vi "Item Setting.vi"(3 "error in":errorcluster) -> (0 "error out":errorcluster)   [LabVIEW 2020]
panel:
  in  "Edit Button":bool
  in  "Delete Button":bool
  in  "Add Button":bool
  in  "Items":i32(listbox)
  in  "Exit Button":bool
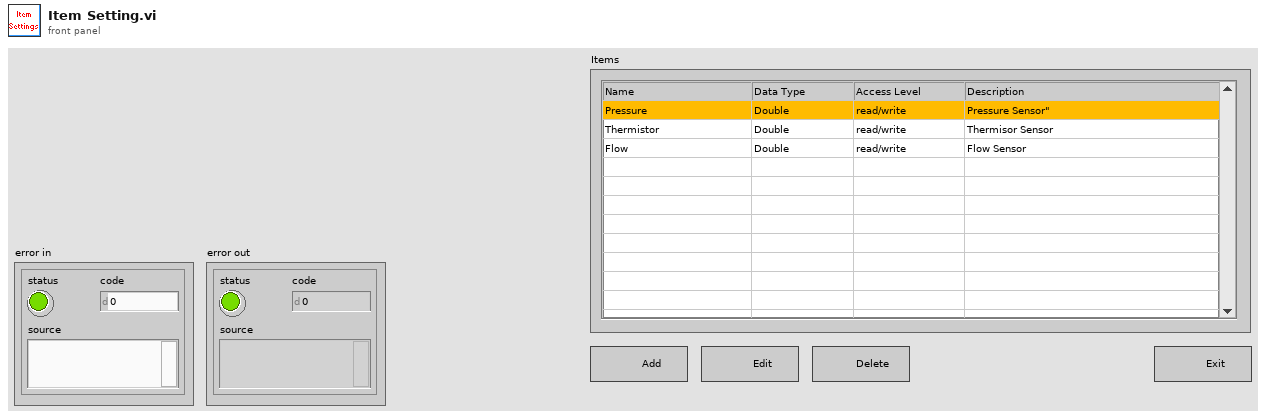
[diagram p1: front panel]
types:
  T1 = cluster{"Name":string, "Data type":u16, "Access level":u16, "Description":string}[]
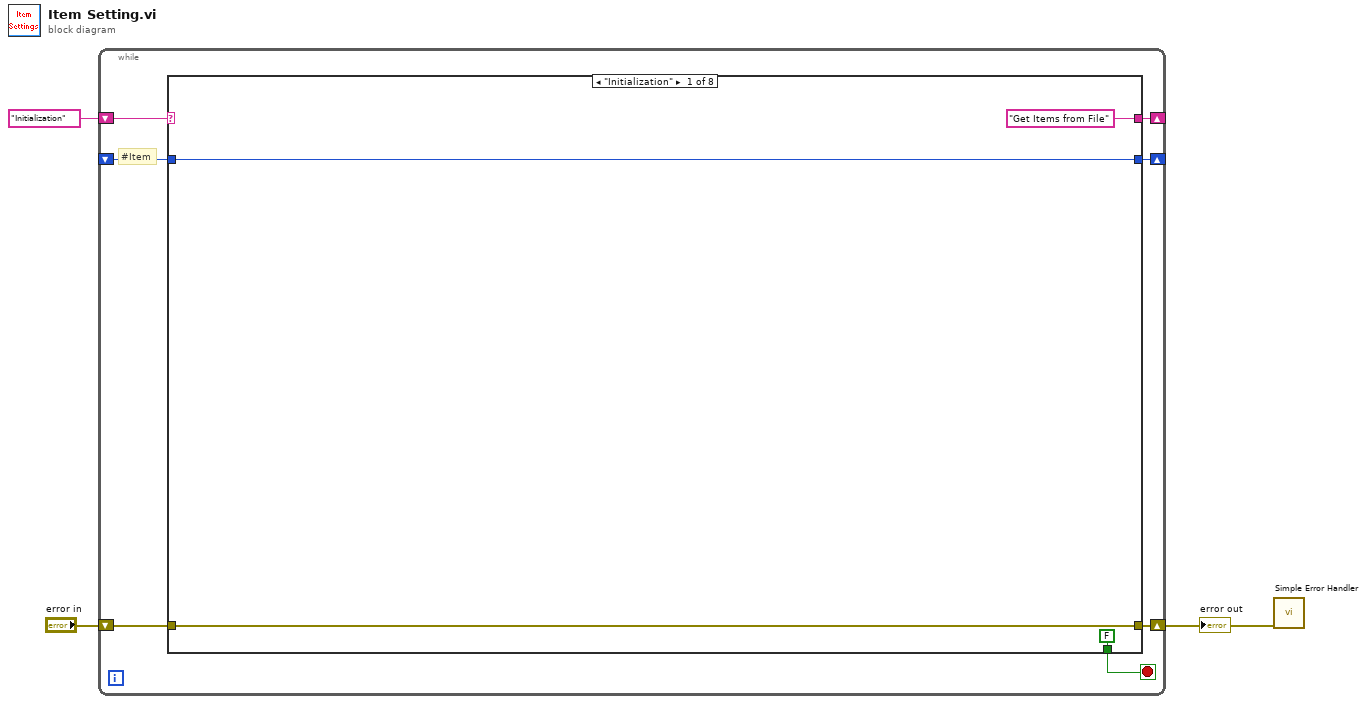
[diagram p0: block diagram]
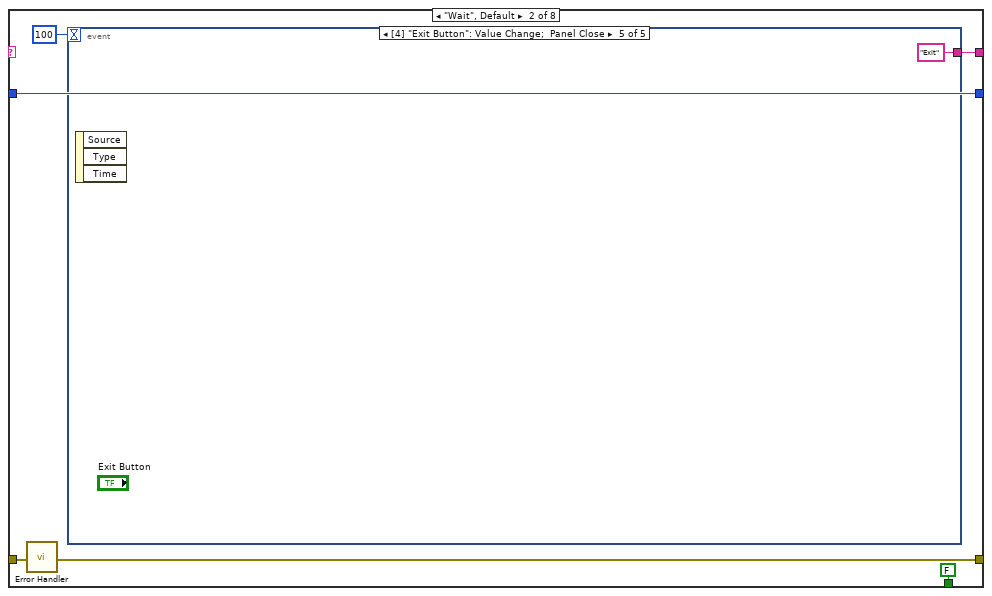
[diagram p2: hidden frame]
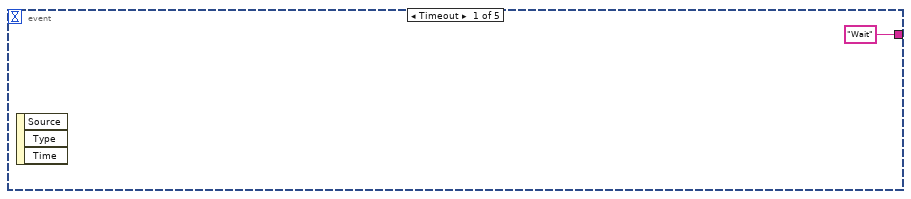
[diagram p3: hidden frame]
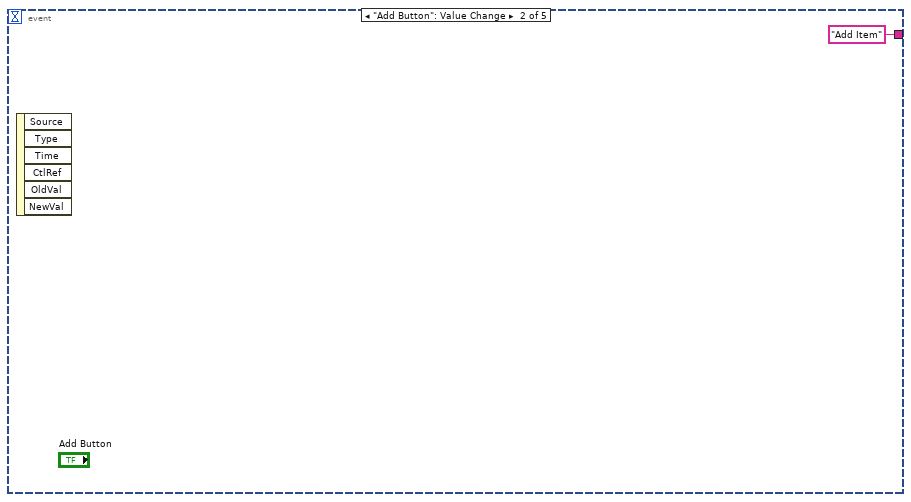
[diagram p4: hidden frame]
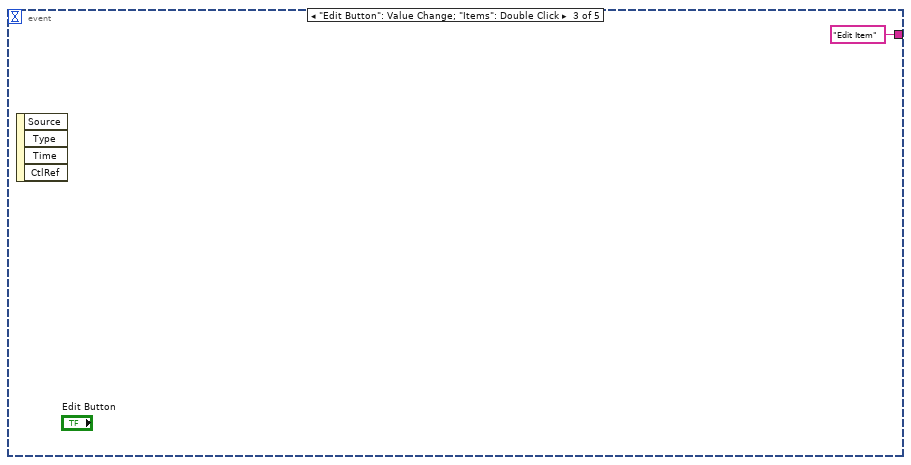
[diagram p5: hidden frame]
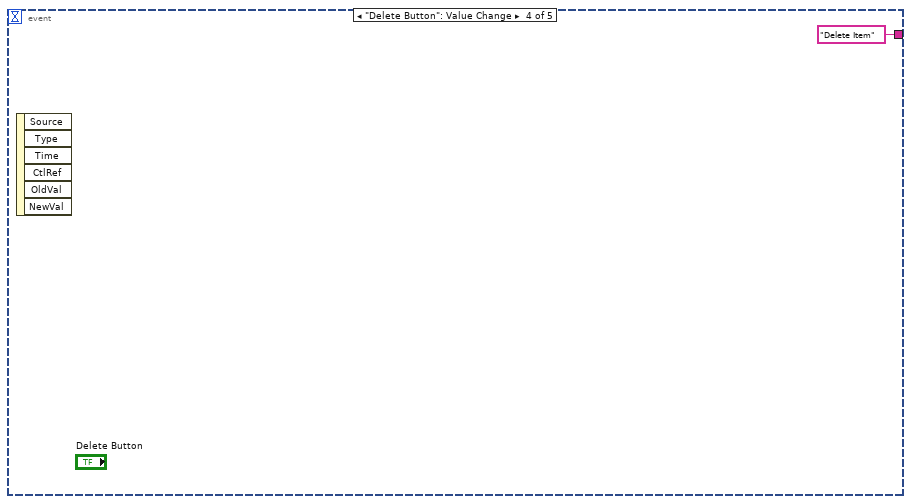
[diagram p6: hidden frame]
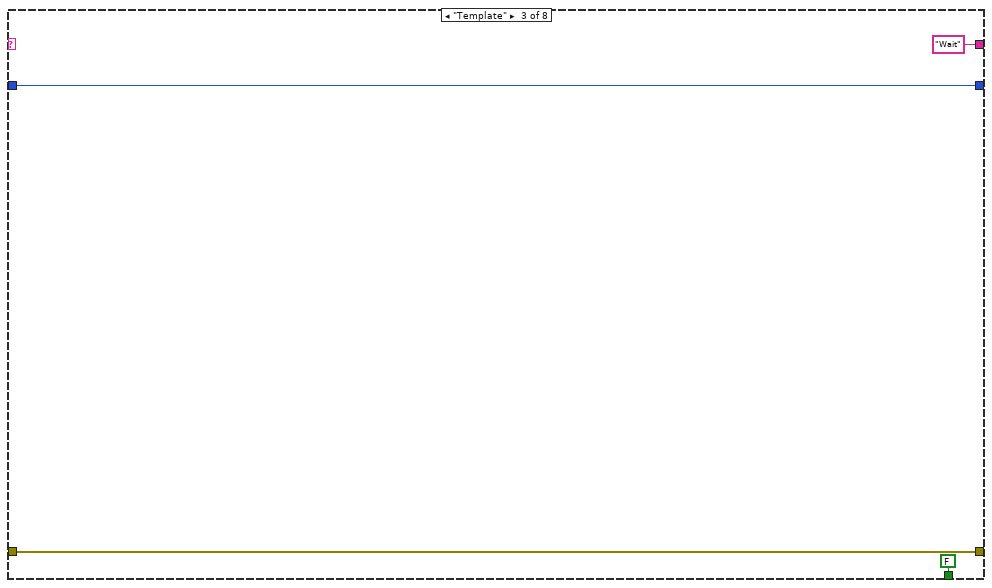
[diagram p7: hidden frame]
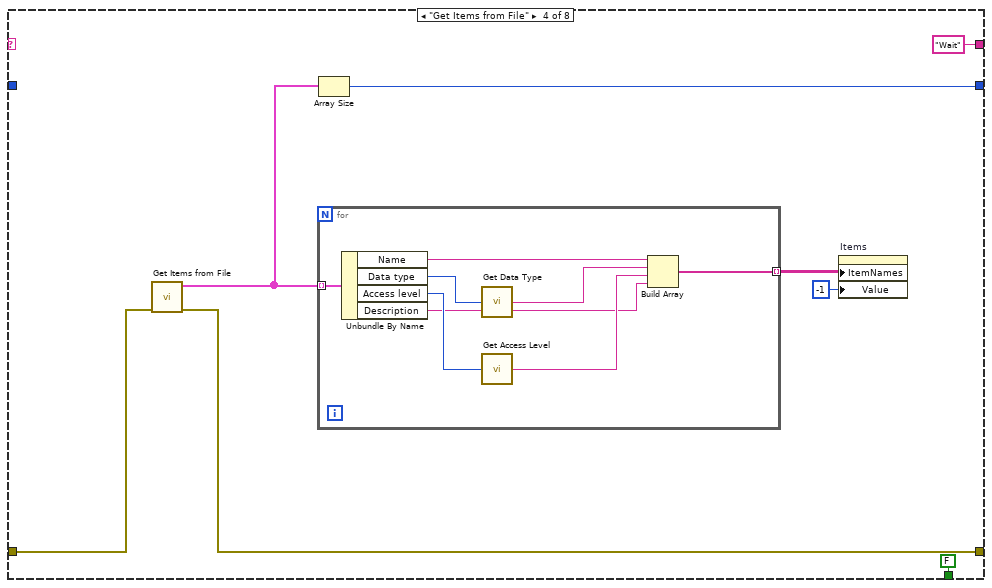
[diagram p8: hidden frame]
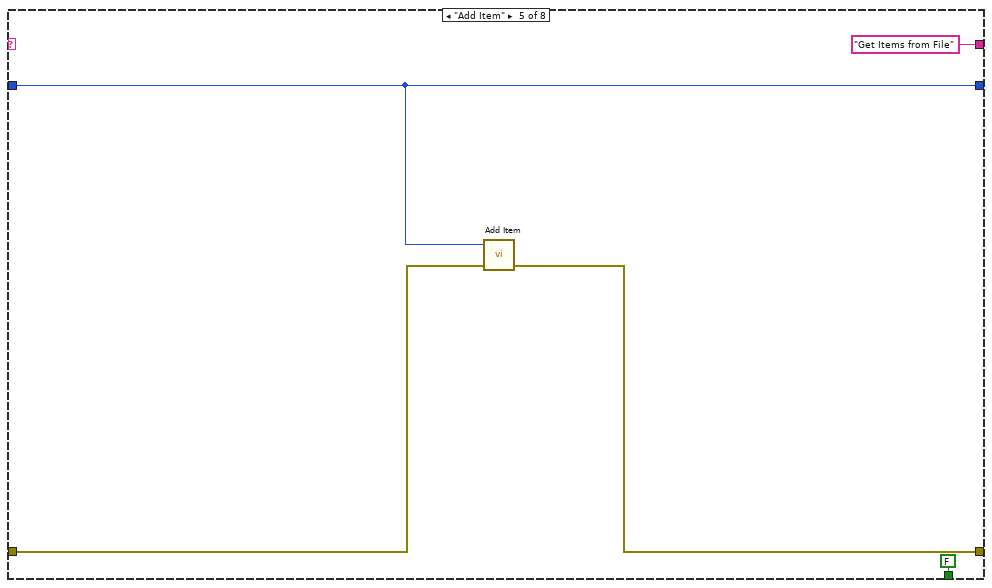
[diagram p9: hidden frame]
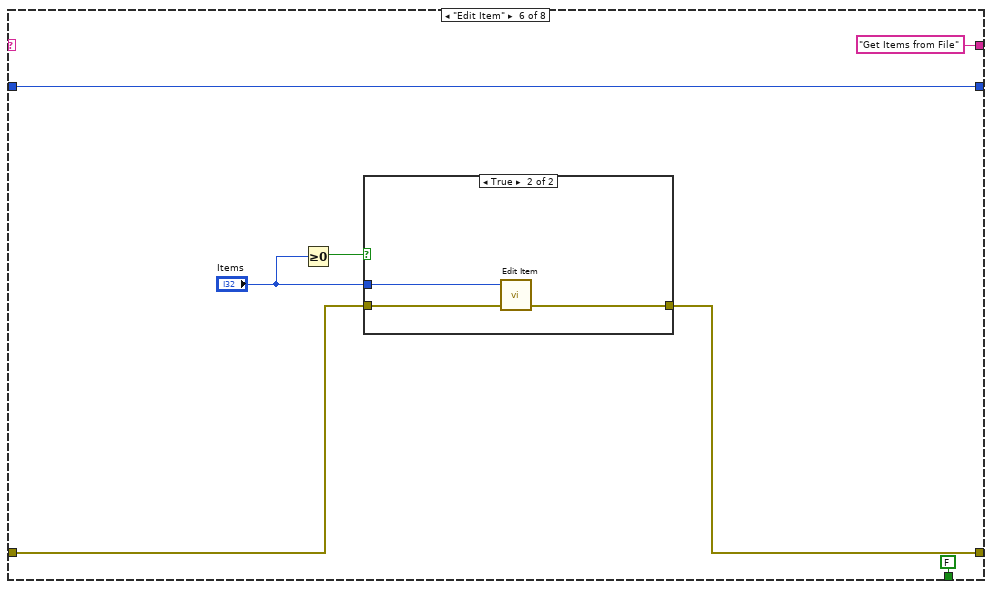
[diagram p10: hidden frame]
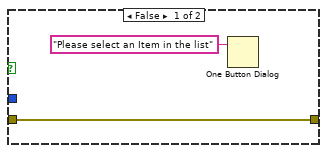
[diagram p11: hidden frame]
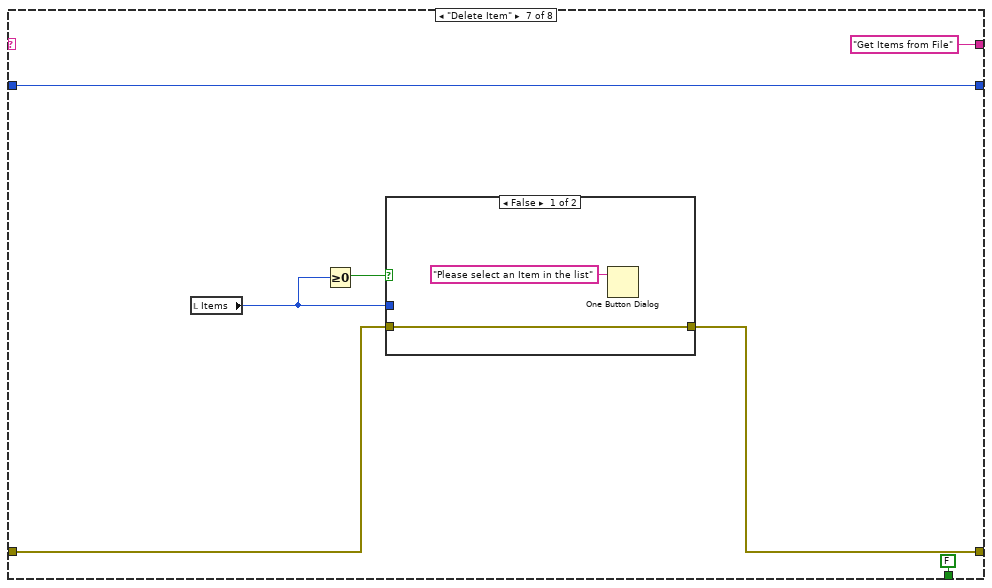
[diagram p12: hidden frame]
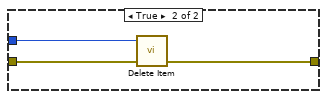
[diagram p13: hidden frame]
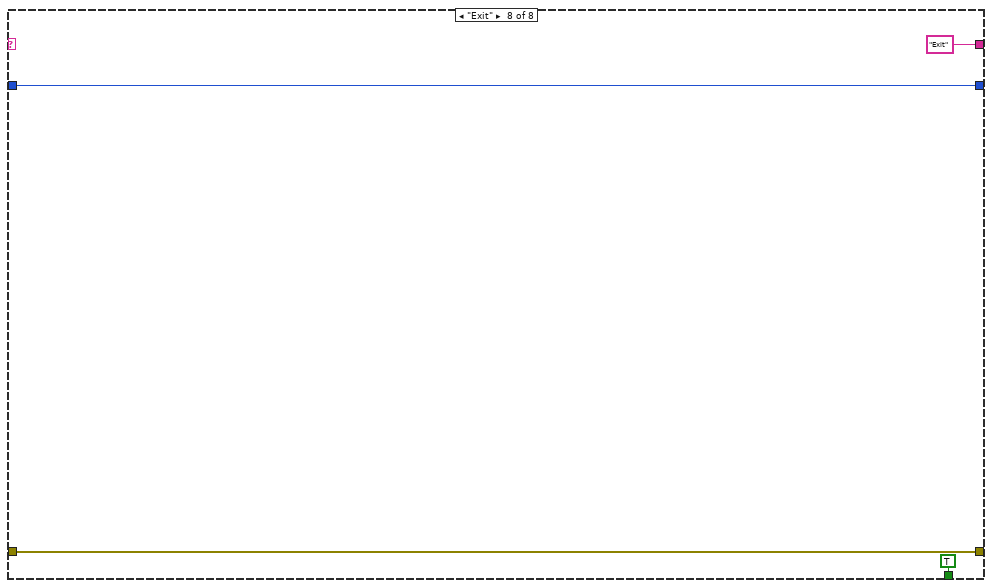
[diagram p14: hidden frame]
diagram:
  n1 = while {
    shift-right: [w9] -> _
    shift-left: "Initialization" -> [w10]
    shift-right: [w6] -> w1
    shift-left: "error in" -> [w7]
    shift-right: [w5] -> _
    shift-left: _ -> [w4]
    stop <- w8 stop-if-true
    # "#Item"
    n2 = case shown="\"Initialization\"" w10 {
      tunnel: ["Get Items from File" w18 "Wait" "Wait" "Get Items from File" "Get Items from File" "Get Items from File" "Exit"] -> w9
      tunnel: [FALSE FALSE FALSE FALSE FALSE FALSE FALSE TRUE] -> w8
      tunnel: w7 -> [w12 w15 w27 w34 w46 w53 w63 w76]
      tunnel: [w12 w16 w27 w35 w47 w54 w64 w76] -> w6
      tunnel: [w11 w17 w26 w32 w48 w55 w67 w75] -> w5
      tunnel: w4 -> [w11 w17 w26 _ w48 w55 w67 w75]
      frame "Initialization" {
      }
      frame "Wait", Default {
        n3 = call "Error Handler.vi"("Error in"=w15) -> ("Error out"=w16:errorcluster)
        n4 = event shown="[4] \"Exit Button\": Value Change;  Panel Close" {
          selector: _ -> [_ _ _ _ _]
          dyn-events: _ -> [_ _ _ _ _]
          timeout: 100 ("ms") -> [_ _ _ _ _]
          tunnel: ["Wait" "Add Item" "Edit Item" "Delete Item" "Exit"] -> w18
          event Timeout {
            n5 = event-data() -> ()  [unwired: 1 in, 3 out]
          }
          event "Add Button": Value Change {
            n6 = event-data() -> ()  [unwired: 1 in, 6 out]
          }
          event "Edit Button": Value Change; "Items": Double Click {
            n7 = event-data() -> ()  [unwired: 1 in, 4 out]
          }
          event "Delete Button": Value Change {
            n8 = event-data() -> ()  [unwired: 1 in, 6 out]
          }
          event "Exit Button": Value Change; Panel Close {
            n9 = event-data() -> ()  [unwired: 1 in, 3 out]
          }
        }
      }
      frame "Template" {
      }
      frame "Get Items from File" {
        n10 = call "Get Items from File.vi"("Error in"=w34) -> ("Error out"=w35:errorcluster, "Items"=w33:T1)  [unwired: 9 in]
        n11 = for {
          tunnel: w33 -> [w43] mode=indexing
          tunnel: [w40] -> w31 mode=indexing
          n12 = Unbundle By Name(w43) -> ("Name"=w42:string, "Data type"=w41:u16, "Access level"=w39:u16, "Description"=w38:string)
          n13 = call "Get Data Type.vi"("Data Type Index"=w41) -> ("Data Type Name"=w45:string)
          n14 = call "Get Access Level.vi"("Access Level Index"=w39) -> ("Access Level Name"=w44:string)
          n15 = Build Array "Build Array"(w42, w45, w44, w38) -> (w40:string[])
        }
        n16 = Array Size(array=w33) -> (size(s)=w32:i32)
        n17 = property on="Items" class="MCListbox (strict)"("ItemNames"=w31, "Value"=-1 ("Items")) -> ()  [unwired: 2 in, 2 out]
      }
      frame "Add Item" {
        n18 = call "Add Item.vi"("Error in"=w46, "Item"=w48) -> ("Error out"=w47:errorcluster)  [unwired: 3 in]
      }
      frame "Edit Item" {
        n19 = Greater Or Equal To 0?(x="Items") -> (x >= 0?=w51:bool)
        n20 = case shown="True" w51 {
          tunnel: [w59 w62] -> w54
          tunnel: w53 -> [w59 w61]
          tunnel: "Items" -> [_ w60]
          frame False {
            n21 = One Button Dialog(message="Please select an Item in the list") -> ()  [unwired: 1 in, 1 out]
          }
          frame True {
            n22 = call "Edit Item.vi"("Error in"=w61, "Item"=w60) -> ("Error out"=w62:errorcluster)  [unwired: 3 in]
          }
        }
      }
      frame "Delete Item" {
        n23 = local read "Items"() -> (w65:i32)
        n24 = Greater Or Equal To 0?(x=w65) -> (x >= 0?=w66:bool)
        n25 = case shown="False" w66 {
          tunnel: w65 -> [_ w74]
          tunnel: w63 -> [w70 w73]
          tunnel: [w70 w72] -> w64
          frame False {
            n26 = One Button Dialog(message="Please select an Item in the list") -> ()  [unwired: 1 in, 1 out]
          }
          frame True {
            n27 = call "Delete Item.vi"("Error in"=w73, "Item"=w74) -> ("Error out"=w72:errorcluster)  [unwired: 3 in]
          }
        }
      }
      frame "Exit" {
      }
    }
  }
  "error out" <- w1
  n28 = call <vilib>:"Simple Error Handler.vi"("error in (no error)"=w1) -> ()  [unwired: 4 in, 5 out]
